vi "Find First Error and Warning.vi"(4 "error in (no error)":errorcluster, 7 "error code":i32) -> (0 "error out":errorcluster, 2 "error?":bool)   [LabVIEW 2017, in "NI_ReportGenerationCore.lvlib"]
uses:
  <vilib>/Utility/NIReport.llb/NI_ReportGenerationCore.lvlib
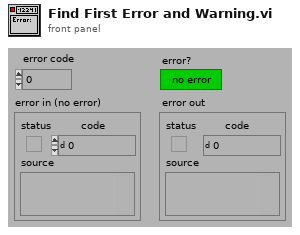
[diagram p1: front panel]
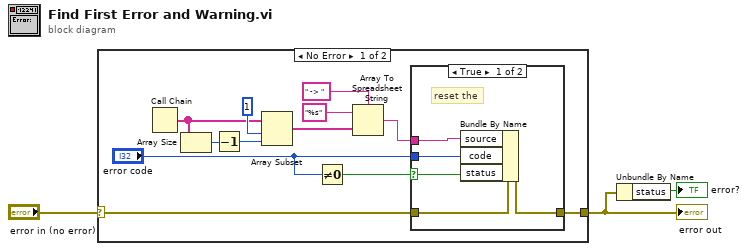
[diagram p0: block diagram]
diagram:
  n1 = case shown="No Error" "error in (no error)" {
    selector: "error in (no error)" -> [w4 w22]
    tunnel: [w15 w22] -> w3
    frame No Error {
      n2 = Call Chain() -> (call chain=w12:string[])
      n3 = Array Size(array=w12) -> (size(s)=w13:i32)
      n4 = Decrement(x=w13) -> (x-1=w11:i32)
      n5 = Array Subset(array=w12, index=1 ("Array Index"), length=w11) -> (w10:string[])
      n6 = Not Equal To 0?(x="error code") -> (x != 0?=w7:bool)
      n7 = Array To Spreadsheet String(delimiter (Tab)=" -> ", array=w10, 3:"%s" ("format string")) -> (spreadsheet string=w6:string)
      n8 = case shown="True" w7 {
        selector: w7 -> [w16 _]
        tunnel: w4 -> [w20 w21]
        tunnel: [w19 w21] -> w15
        tunnel: "error code" -> [w18 _]
        tunnel: w6 -> [w17 _]
        frame True {
          # "reset the"
          n9 = Bundle By Name(cluster=w20, "source"=w17, "code"=w18, "status"=w16) -> (w19:errorcluster)
        }
        frame False {
        }
      }
    }
    frame Error {
    }
  }
  "error out" <- w3
  n10 = Unbundle By Name(w3) -> ("status"=→"error?":bool)
